vi "RTMain.ReadWrite Data.vi"(8 "error in":errorcluster, 9 "ReadUpdate":refnum<k33>, 10 "Write to VS Engine FIFO":refnum<k33>, 11 "Data Refs":T1 {"Write Refs" format="%.0x"; "Read Refs" format="%.0x"}) -> (0 "error out":errorcluster, 2 "Read Occured":bool, 3 "Data Refs":T1 {"Write Refs" format="%.0x"; "Read Refs" format="%.0x"})   [LabVIEW 2017, in "OPC UA Client Engine.lvlib"]
uses:
  OPC UA Client Engine.lvlib
  Shared/Tags.ReadWriteRefs.ctl
  <vilib>/NI Veristand/Custom Device API/Data Reference.ctl
  <vilib>/NI Veristand/Custom Device API/Global Data Refs.vi
  <vilib>/NI VeriStand/Custom Device API/Custom Device API.lvlib
  Shared/OPC UA Client Shared.lvlib
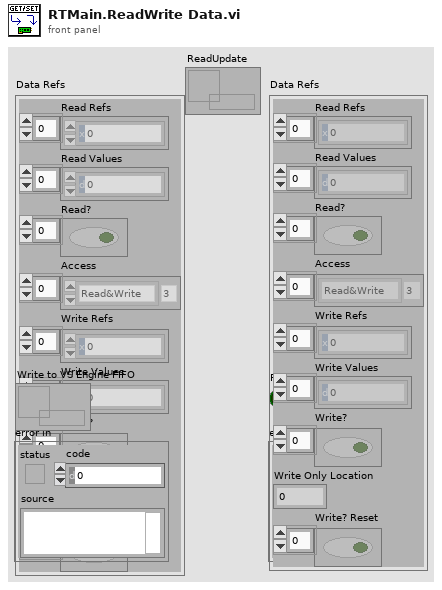
[diagram p1: front panel]
types:
  T1 = typedef "OPC UA Client Shared.lvlib/Tags.ReadWriteRefs.ctl" = cluster{"Read Refs":T2[], "Read Values":dbl[], "Read?":bool[], "Access":enum8{"Null", "Read", "Write", "Read&Write"}[], "Write Refs":T2[], "Write Values":dbl[], "Write?":bool[], "Write Only Location":u32, "Write? Reset":bool[]}
  T2 = typedef "Custom Device API.lvlib/Data Reference.ctl" = i32
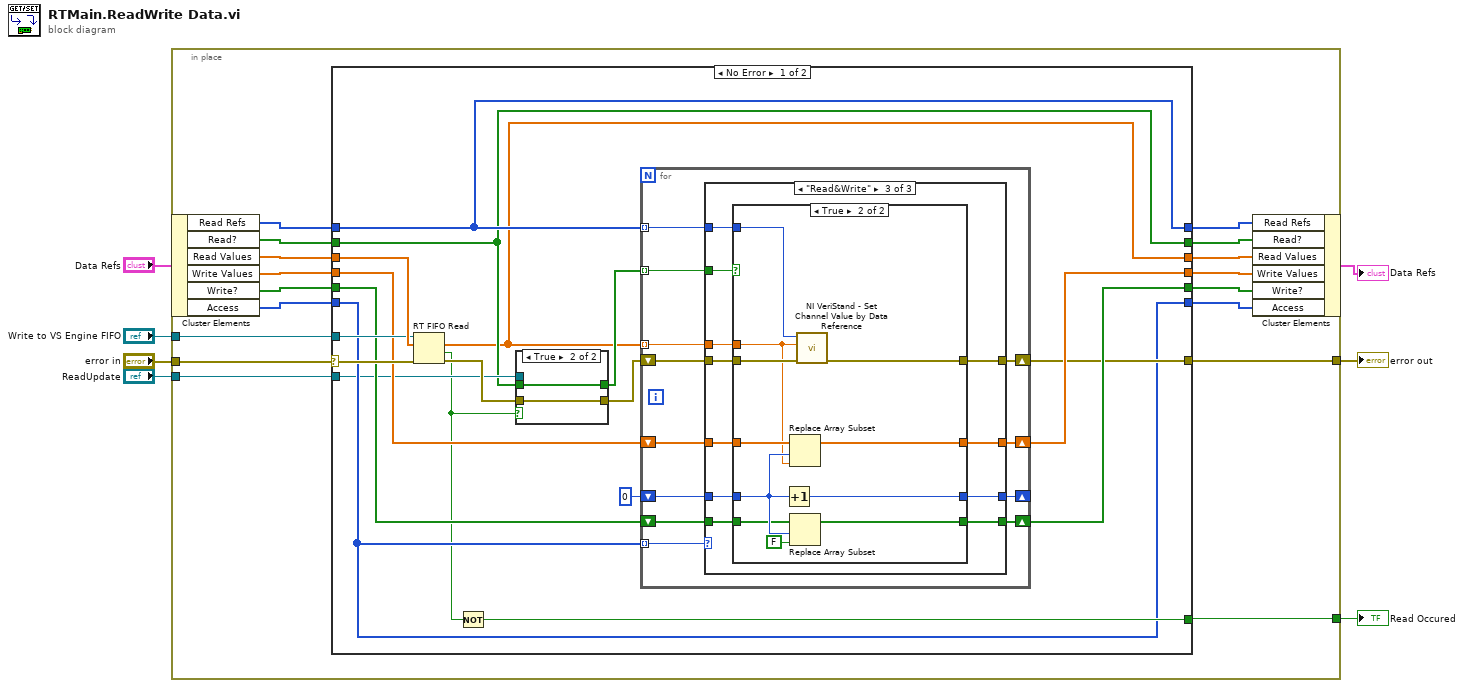
[diagram p0: block diagram]
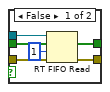
[diagram p2: hidden frame]
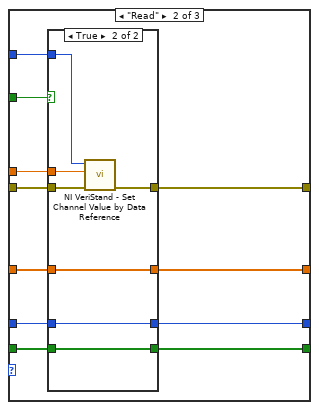
[diagram p4: hidden frame]
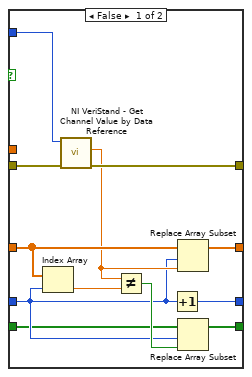
[diagram p6: hidden frame]
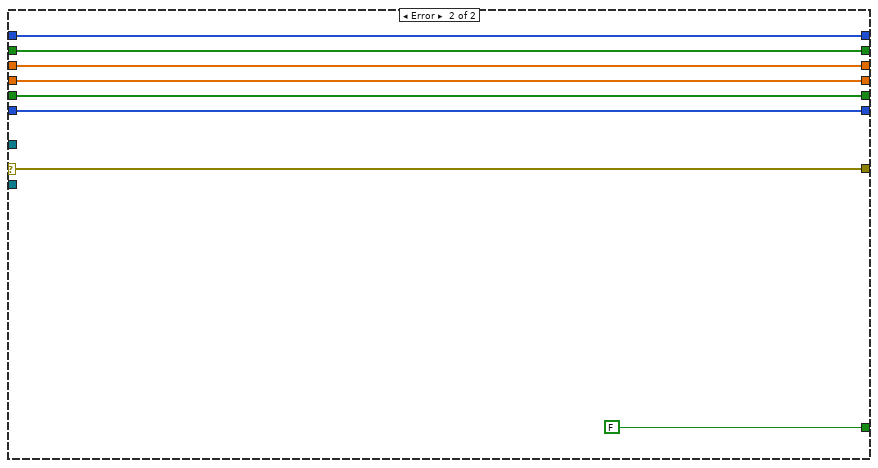
[diagram p7: hidden frame]
diagram:
  n1 = in-place {
    in-place-border: [w24] -> w7
    in-place-border: [w23] -> w6
    in-place-border: "error in" -> [w18]
    in-place-border: "Write to VS Engine FIFO" -> [w17]
    in-place-border: "ReadUpdate" -> [w9]
    n2 = in-place-cluster #1("Data Refs") -> ("Read Refs"=w22:T2[], "Read?"=w10:bool[], "Read Values"=w21:dbl[], "Write Values"=w16:dbl[], "Write?"=w14:bool[], "Access"=w12:enum8{"Null", "Read", "Write", "Read&Write"}[])
    n3 = case shown="No Error" w18 {
      selector: w18 -> [w43 w131]
      tunnel: [w34 w131] -> w24
      tunnel: [w25 w129] -> w20
      tunnel: [w42 FALSE ("C Read Occured?")] -> w23
      tunnel: w22 -> [w40 w128]
      tunnel: w21 -> [w41 w129]
      tunnel: [w40 w128] -> w19
      tunnel: w17 -> [w39 _]
      tunnel: w12 -> [w33 w125]
      tunnel: w16 -> [w38 w127]
      tunnel: [w36 w127] -> w15
      tunnel: w14 -> [w37 w126]
      tunnel: [w35 w126] -> w13
      tunnel: [w33 w125] -> w11
      tunnel: w10 -> [w30 w124]
      tunnel: w9 -> [w31 _]
      tunnel: [w30 w124] -> w8
      frame No Error {
        n4 = RT FIFO Read(0:w39, 1:w41, 3:w43) -> (9:w25:dbl[], 10:w26:bool, 11:w32:errorcluster)  [unwired: 1 in, 2 out]
        n5 = Not(x=w26) -> (.not. x?=w42:bool)
        n6 = case shown="True" w26 {
          tunnel: w32 -> [w49 w51]
          tunnel: w31 -> [w48 _]
          tunnel: w30 -> [w47 w50]
          tunnel: [w46 w51] -> w28
          tunnel: [w45 w50] -> w27
          frame False {
            n7 = RT FIFO Read(0:w48, 1:w47, 2:1 ("timeout in ms (0)"), 3:w49) -> (9:w45:bool[], 11:w46:errorcluster)  [unwired: 3 out]
          }
          frame True {
          }
        }
        n8 = for {
          shift-right: [w63] -> w34
          shift-left: w28 -> [w62]
          tunnel: w40 -> [w60] mode=indexing
          tunnel: w33 -> [w53] mode=indexing
          shift-right: [w58] -> _
          shift-left: u32 0 -> [w57]
          shift-right: [w56] -> w36
          shift-left: w38 -> [w59]
          shift-right: [w54] -> w35
          shift-left: w37 -> [w55]
          tunnel: w27 -> [w52] mode=indexing
          tunnel: w25 -> [w61] mode=indexing
          n9 = case shown="\"Read&Write\"" w53 {
            tunnel: [w64 w78 w100] -> w63
            tunnel: w62 -> [w64 w77 w99]
            tunnel: w61 -> [_ w76 w98]
            tunnel: w60 -> [_ w75 w97]
            tunnel: w52 -> [_ w74 w96]
            tunnel: w59 -> [w65 w73 w95]
            tunnel: [w67 w72 w94] -> w58
            tunnel: w57 -> [w67 w71 w93]
            tunnel: [w65 w70 w92] -> w56
            tunnel: w55 -> [w66 w69 w91]
            tunnel: [w66 w68 w90] -> w54
            frame "Null", Default {
            }
            frame "Read" {
              n10 = case shown="True" w74 {
                tunnel: w76 -> [_ w83]
                tunnel: [w82 w88] -> w78
                tunnel: w77 -> [w82 w89]
                tunnel: w75 -> [_ w87]
                tunnel: w73 -> [w80 w86]
                tunnel: [w81 w85] -> w72
                tunnel: w71 -> [w81 w85]
                tunnel: [w80 w86] -> w70
                tunnel: w69 -> [w79 w84]
                tunnel: [w79 w84] -> w68
                frame False {
                }
                frame True {
                  n11 = call <vilib>:"NI VeriStand - Set Channel Value by Data Reference.vi"("error in (no error)"=w89, "Value"=w83, "Data Reference in"=w87) -> ("error out"=w88:errorcluster)  [unwired: 8 in]
                }
              }
            }
            frame "Read&Write" {
              n12 = case shown="True" w96 {
                tunnel: w98 -> [_ w113]
                tunnel: [w110 w122] -> w100
                tunnel: w99 -> [w111 w123]
                tunnel: w97 -> [w112 w121]
                tunnel: w95 -> [w107 w120]
                tunnel: [w109 w117] -> w94
                tunnel: w93 -> [w103 w119]
                tunnel: [w108 w118] -> w92
                tunnel: w91 -> [w102 w116]
                tunnel: [w101 w115] -> w90
                frame False {
                  n13 = Index Array(array=w107, index=w103) -> (element=w104:dbl)
                  n14 = call <vilib>:"NI VeriStand - Get Channel Value by Data Reference.vi"("error in (no error)"=w111, "Data Reference in"=w112) -> ("error out"=w110:errorcluster, "Value"=w105:dbl)  [unwired: 8 in]
                  n15 = Not Equal?(x=w105, y=w104) -> (x != y?=w106:bool)
                  n16 = Increment(x=w103) -> (x+1=w109:u32)
                  n17 = Replace Array Subset(array=w107, new element=w105, index=w103) -> (w108:dbl[])
                  n18 = Replace Array Subset(array=w102, new element=w106, index=w103) -> (w101:bool[])
                }
                frame True {
                  n19 = Increment(x=w119) -> (x+1=w117:u32)
                  n20 = Replace Array Subset(array=w120, new element=w113, index=w119) -> (w118:dbl[])
                  n21 = Replace Array Subset(array=w116, new element=FALSE ("new element/subarray"), index=w119) -> (w115:bool[])
                  n22 = call <vilib>:"NI VeriStand - Set Channel Value by Data Reference.vi"("error in (no error)"=w123, "Value"=w113, "Data Reference in"=w121) -> ("error out"=w122:errorcluster)  [unwired: 8 in]
                }
              }
            }
          }
        }
      }
      frame Error {
      }
    }
    n23 = in-place-cluster #1("Read Refs"=w19, "Read?"=w8, "Read Values"=w20, "Write Values"=w15, "Write?"=w13, "Access"=w11) -> (→"Data Refs":T1)
  }
  "error out" <- w7
  "Read Occured" <- w6
